vi "Get Current GPS Location.vi"() -> (0 "True":bool)   [LabVIEW 2011]
uses:
  _GlobalVariables&Libraries/ATV Program Global Variables.vi
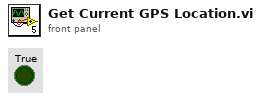
[diagram p1: front panel]
types:
  T1 = cluster{"GPS VISA resource name":refnum<visa-resource-name>, "GPS Error":errorcluster, "Disable GPS VISA":bool, "Latitude":dbl, "Longitude":dbl, "Latitude Uncertainty":dbl, "Longitude Uncertainty":dbl, "GPS Signal":u32}
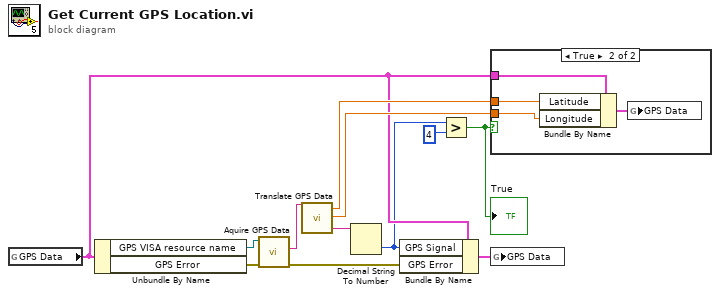
[diagram p0: block diagram]
diagram:
  n1 = global read "ATV Program Global Variables.vi" "GPS Data"() -> (w4:T1)
  n2 = Unbundle By Name(w4) -> ("GPS VISA resource name"=w11:refnum<visa-resource-name>, "GPS Error"=w2:errorcluster)
  n3 = call "Aquire GPS Data.vi"("error in"=w2, "VISA resource name in"=w11) -> ("error out"=w1:errorcluster, "read buffer"=w12:string)  [unwired: 7 in, 1 out]
  n4 = call "Translate GPS Data.vi"("Read Buffer"=w12) -> ("Latitude"=w10:dbl, "Longitude"=w9:dbl, "Satellites Tracked"=w8:string)  [unwired: 19 in, 5 out]
  n5 = Decimal String To Number(string=w8) -> (number=w3:i32)  [unwired: 2 in, 1 out]
  n6 = Bundle By Name(cluster=w4, "GPS Signal"=w3, "GPS Error"=w1) -> (w5:T1)
  n7 = Greater?(x=w3, y=4) -> (0:w6:bool)
  "True" <- w6
  n8 = case shown="True" w6 {
    tunnel: w4 -> [_ w15]
    tunnel: w10 -> [_ w14]
    tunnel: w9 -> [_ w13]
    frame False {
    }
    frame True {
      n9 = Bundle By Name(cluster=w15, "Latitude"=w14, "Longitude"=w13) -> (w16:T1)
      n10 = global write "ATV Program Global Variables.vi" "GPS Data"(w16) -> ()
    }
  }
  n11 = global write "ATV Program Global Variables.vi" "GPS Data"(w5) -> ()
